vi "ANSI - Fractional-octave Analysis.vi"(0 "scaled signal [EU]":dbl[](array[numeric]) format="%.2f", 1 "sampling frequency [Hz]":dbl=10000.0 format="%.2f", 2 "bandwidth":T5(ring)=enum."1/3 octave", 3 "frequency range [Hz]":cluster{"low freq.":dbl, "high freq.":dbl}={"low freq."=125.0, "high freq."=8000.0} {"high freq." min=0.001 format="%.2f"; "low freq." min=0.001 format="%.2f"}, 4 "dB On (T)":bool=TRUE, 5 "channel info":T1={"sensor sensitivity [mV/EU]"=1000.0, "engineering units"=1, "dB reference [EU]"=1.0, "custom label"="EU", "weighting filter"=0, "pregain [dB]"=0.0} {"pregain [dB]" format="%.2f"; "weighting filter" items=["Linear", "A-weighting", "B-weighting", "C-weighting", "ITU-R 468-4", "Dolby", "CCITT", "C-message"]; "dB reference [EU]" format="%^.1e"; "engineering units" items=["custom..."=0, "V"=1, "A"=21, "Pa"=2, "N"=20, "g"=3, "m/s^2"=4, "m/s"=5, "m"=6, "mm/s"=12, "mm"=13, "microns/s"=14, "microns"=15, "in/s^2"=7, "in/s"=8, "in"=9, "mils/s"=10, "mils"=11, "rad/s^2"=16, "rad/s"=17, "rad"=18, "strain"=19]; "sensor sensitivity [mV/EU]" format="%.2f"}, 6 "averaging type":T7(ring)=enum."Exponential", 7 "filter init/cont (init:F)":bool, 8 "averaging parameters":T4={"linear mode"=enum."start averaging once settled", "exponential mode"=enum."Fast", "time constant [ms]"=125.0, "confidence [dB]"=1.0, "peak mode"=enum."start peak detection once settled"} {"confidence [dB]" min=0.01 max=10.0 format="%.2f"; "time constant [ms]" min=0.0 format="%.2f"}, 9 "reset averaging (F)":bool) -> (12 "nominal frequencies (string)":string[](array[string]), 13 "bandedge frequencies [Hz]":T6(array[cluster]) {"midband" format="%.2f"; "f high" format="%.2f"; "f low" format="%.2f"}, 14 "band power [dB EU]":dbl[](array[numeric]) format="%.2f", 15 "unit label":string, 16 "nominal frequencies [Hz]":dbl[](array[numeric]) format="%.2f", 17 "total band power [dB EU]":dbl format="%.2f", 18 "settled?":bool, 19 "error":bool)   [LabVIEW 2017]
doc: "Performs a fractional-octave analysis on the input signal. The fractional-octave filters are designed in accordance with ANSI S1.11-1986, Order 3, Type 1-D, optional range. To meet this standard, the sampling frequency must be at least 3 times the highest midband frequency for octave analysis and at least 2.5 times the highest midband frequency for 1/3, 1/6, 1/12, or 1/24 octave analysis.\nAvailable averaging types are Linear, Exponential (default), Equal confidence, and Peak. Based on the selected averaging type, this VI uses the additional settings in averaging parameters.\nThis VI returns the power in each fractional-octave band and the total band power, both expressed in decibels. The total band power is defined as the sum of the individual band powers.\nTo ensure a continuous filtering operation call this VI the first time with filter init/cont set to FALSE and then call it with filter init/cont set to TRUE."
uses:
  <vilib>/addons/Sound and Vibration/compatibility/Controls/svl_Channel Info.ctl
  <vilib>/addons/Sound and Vibration/compatibility/Controls/svl_Engineering Units Text Ring.ctl
  <vilib>/addons/Sound and Vibration/compatibility/Controls/svl_Weighting Filter Text Ring.ctl
  <vilib>/addons/_NISVFA/_Shared subVIs/Controls/svc_Octave Standard.ctl
  <vilib>/addons/Sound and Vibration/svt_Octave/SoundVib_Octave.lvlib
panel:
  # "Linear"
  # "Exponential"
  # "Equal confidence"
  # "Peak"
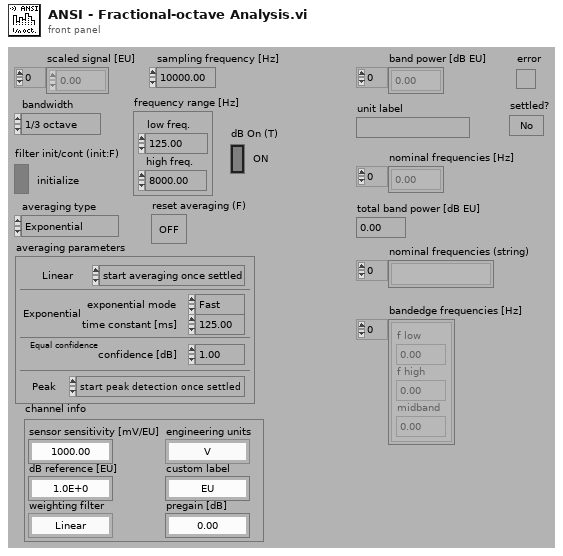
[diagram p1: front panel]
types:
  T1 = typedef "svl_Channel Info.ctl" = cluster{"sensor sensitivity [mV/EU]":dbl, "engineering units":T2, "dB reference [EU]":dbl, "custom label":string, "weighting filter":T3, "pregain [dB]":dbl}
  T2 = typedef "svl_Engineering Units Text Ring.ctl" = u16
  T3 = typedef "svl_Weighting Filter Text Ring.ctl" = u16
  T4 = cluster{"linear mode":enum16{"start averaging once settled", "continuous averaging", "single averaging"}, "exponential mode":enum16{"Slow", "Fast", "Impulse", "Custom"}, "time constant [ms]":dbl, "confidence [dB]":dbl, "peak mode":enum16{"start peak detection once settled", "continuous peak detection", "single peak detection"}}
  T5 = enum16{"1 octave", "1/3 octave", "1/6 octave", "1/12 octave", "1/24 octave"}
  T6 = cluster{"f low":dbl, "f high":dbl, "midband":dbl}[]
  T7 = enum16{"Linear", "Exponential", "Equal confidence", "Peak"}
  T8 = typedef "svc_Octave Standard.ctl" = enum16{"ANSI S1.11", "IEC 61260"}
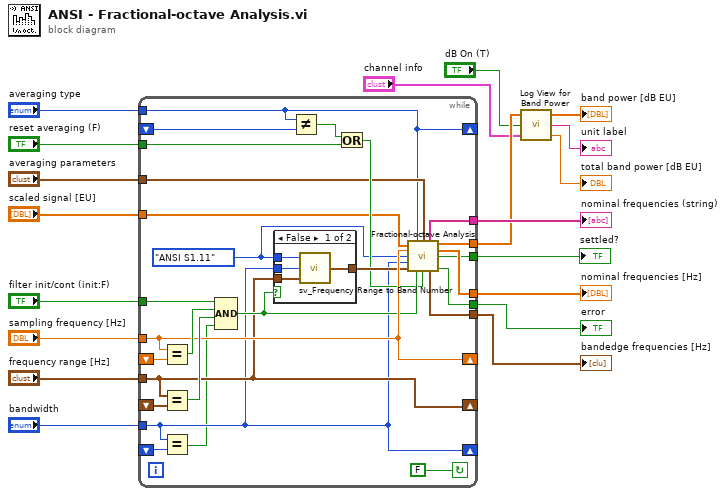
[diagram p0: block diagram]
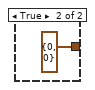
[diagram p2: hidden frame]
diagram:
  n1 = while {
    tunnel: "scaled signal [EU]" -> [w21]
    tunnel: "averaging parameters" -> [w25]
    tunnel: "reset averaging (F)" -> [w26]
    tunnel: "averaging type" -> [w24]
    shift-left: _ -> [w29]
    shift-right: [w28] -> _
    tunnel: "bandwidth" -> [w28]
    shift-left: _ -> [w23]
    shift-right: [w24] -> _
    tunnel: [w33] -> w13
    tunnel: [w35] -> w14
    tunnel: [w34] -> w15
    tunnel: [w36] -> w16
    tunnel: [w37] -> w17
    tunnel: [w38] -> w10
    tunnel: "sampling frequency [Hz]" -> [w41]
    shift-left: _ -> [w45]
    shift-right: [w41] -> _
    tunnel: "frequency range [Hz]" -> [w30]
    shift-left: _ -> [w46]
    shift-right: [w30] -> _
    tunnel: "filter init/cont (init:F)" -> [w44]
    stop <- FALSE continue-if-true
    w22 = svc_Octave_Standard."ANSI S1.11" ("Standard")
    n2 = Equal?(x=w41, y=w45) -> (x = y?=w42:bool)
    n3 = Equal?(x=w30, y=w46) -> (x = y?=w43:bool)
    n4 = Equal?(x=w28, y=w29) -> (x = y?=w27:bool)
    n5 = Compound Arithmetic op=AND(w44, w42, w43, w27) -> (w40:bool)
    n6 = case shown="False" w40 {
      tunnel: [w50 cluster{"Low band":i32, "High band":i32} {"Low band"=0, "High band"=0} ("Band number")] -> w39
      tunnel: w30 -> [w49 _]
      tunnel: w28 -> [w48 _]
      tunnel: w22 -> [w47 _]
      frame False {
        n7 = call <vilib>:"sv_Frequency Range to Band Number.vi"("frequency range [Hz]"=w49, "bandwidth"=w48, "standard"=w47) -> ("band number"=w50:cluster{"low band":i32, "high band":i32})
      }
      frame True {
      }
    }
    n8 = Not Equal?(x=w24, y=w23) -> (x != y?=w32:bool)
    n9 = Or(x=w32, y=w26) -> (x .or. y?=w31:bool)
    n10 = call <vilib>:"Fractional-octave Analysis.vi"("scaled signal [EU]"=w21, "averaging type"=w24, "averaging parameters"=w25, "sampling frequency [Hz]"=w41, "standard"=w22, "bandwidth"=w28, "band number"=w39, "filter init/cont (init:F)"=w40, "reset averaging (F)"=w31) -> ("nominal frequencies (string)"=w36:string[], "band power [EU^2 rms]"=w38:dbl[], "nominal frequencies [Hz]"=w37:dbl[], "settled?"=w34:bool, "bandedge frequencies [Hz]"=w35:T6, "error"=w33:bool)  [unwired: 1 in]
  }
  "error" <- w13
  "nominal frequencies [Hz]" <- w17
  "settled?" <- w15
  "nominal frequencies (string)" <- w16
  "bandedge frequencies [Hz]" <- w14
  n11 = call <vilib>:"Log View for Band Power.vi"("channel info"="channel info", "dB On (T)"="dB On (T)", "band power [EU^2 rms]"=w10) -> ("total band power [dB EU]"=→"total band power [dB EU]":dbl, "unit label"=→"unit label":string, "log view band power [dB EU]"=→"band power [dB EU]":dbl[])
